vi "测试加减法.vi"() -> ()   [LabVIEW 2011]
uses:
  <vilib>/vision/NI_Vision_Development_Module.lvlib
panel:
  out "Image Pixels (Float)":sgl[][](array[numeric]) format="%.2f"
  out "Image":T1(plugin-control)
  in  "数组 2":i32[][](array[numeric])
  in  "数组":i32[][](array[numeric])
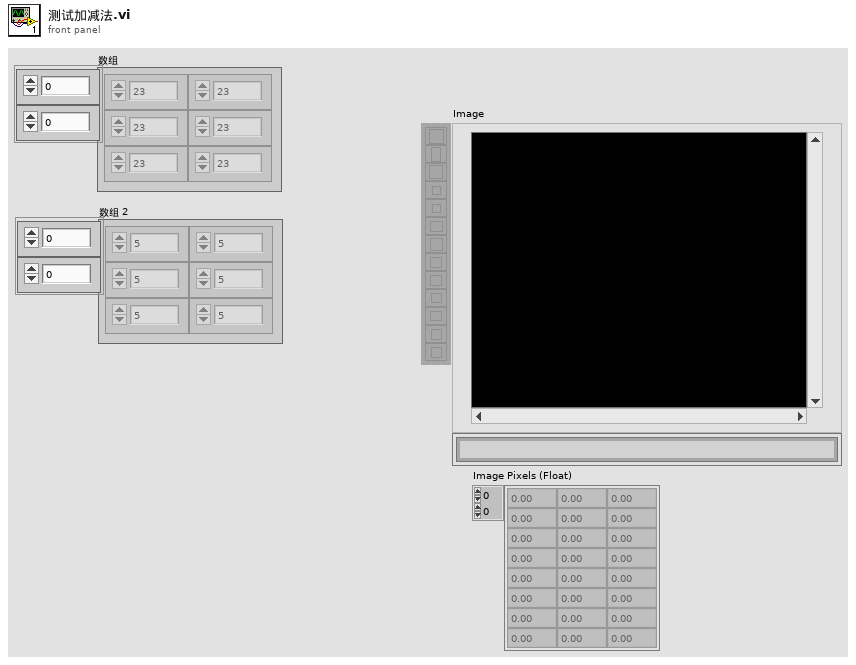
[diagram p1: front panel]
types:
  T1 = typedef "IMAQ Image.ctl" = refnum<image>
  T2 = typedef "Image Type" = u32
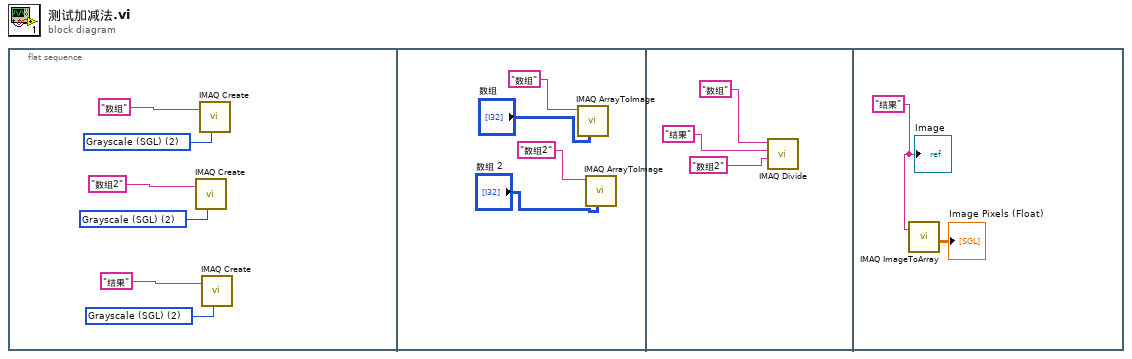
[diagram p0: block diagram]
diagram:
  n1 = flat-sequence {
    frame #0 {
      w1 = T2 2 items=["Grayscale (U8)", "Grayscale (I16)", "Grayscale (SGL)", "Complex (CSG)", "RGB (U32)", "HSL (U32)", "RGB (U64)", "Grayscale (U16)"] ("Image Type")
      w4 = T2 2 items=["Grayscale (U8)", "Grayscale (I16)", "Grayscale (SGL)", "Complex (CSG)", "RGB (U32)", "HSL (U32)", "RGB (U64)", "Grayscale (U16)"] ("Image Type")
      w5 = T2 2 items=["Grayscale (U8)", "Grayscale (I16)", "Grayscale (SGL)", "Complex (CSG)", "RGB (U32)", "HSL (U32)", "RGB (U64)", "Grayscale (U16)"] ("Image Type")
      n2 = call "IMAQ Create"("Image Name"="数组2", "Image Type"=w4) -> ()  [unwired: 3 in, 2 out]
      n3 = call "IMAQ Create"("Image Name"="数组", "Image Type"=w5) -> ()  [unwired: 3 in, 2 out]
      n4 = call "IMAQ Create"("Image Name"="结果", "Image Type"=w1) -> ()  [unwired: 3 in, 2 out]
    }
    frame #1 {
      n5 = call "IMAQ ArrayToImage"("Image Pixels (Float)"="数组", "Image"="数组" ("Image Name")) -> ()  [unwired: 8 in, 2 out]
      n6 = call "IMAQ ArrayToImage"("Image Pixels (Float)"="数组 2", "Image"="数组2" ("Image Name")) -> ()  [unwired: 8 in, 2 out]
    }
    frame #2 {
      n7 = call "IMAQ Divide"("Image Src A"="数组" ("Image Name"), "Image Dst"="结果" ("Image Name"), "Image Src B"="数组2" ("Image Name")) -> ()  [unwired: 4 in, 2 out]
    }
    frame #3 {
      w15 = "结果" ("Image Name")
      n8 = call "IMAQ ImageToArray"("Image"=w15) -> ("Image Pixels (Float)"=→"Image Pixels (Float)":sgl[][])  [unwired: 3 in, 4 out]
      "Image" <- w15
    }
  }
